vi "Handle LogRec.vi"(8 "error in":errorcluster, 10 "LogRecord":refnum<class "LogRecord.lvclass">, 11 "FileHandler in":refnum<class "FileHandler.lvclass">) -> (0 "error out":errorcluster, 3 "FileHandler out":refnum<class "FileHandler.lvclass">)   [LabVIEW 2024, in "hse-logger.lvlib" / "FileHandler.lvclass"]
doc: "Handles the incoming ``LogRecord`` object. If the level of the record is greater or equal to the level of the handler, then the record is written to the file. \n\n____\nHAMPEL SOFTWARE ENGINEERING v2.2.2 (2025-01-16 15:41)"
uses:
  <vilib>/Hampel Software Engineering/HSE Logger/Handler/FileHandler/FileHandler.lvclass
  <vilib>/Hampel Software Engineering/HSE Logger/LogRecord/LogRecord.lvclass
  <vilib>/Hampel Software Engineering/HSE Logger/LogRecord/LogRecord.lvclass/LogRecord.ctl
  <vilib>/Hampel Software Engineering/HSE Logger/Handler/FileHandler/FileHandler.lvclass/FileHandler.ctl
  <vilib>/Hampel Software Engineering/HSE Logger/Formatter/Formatter.lvclass
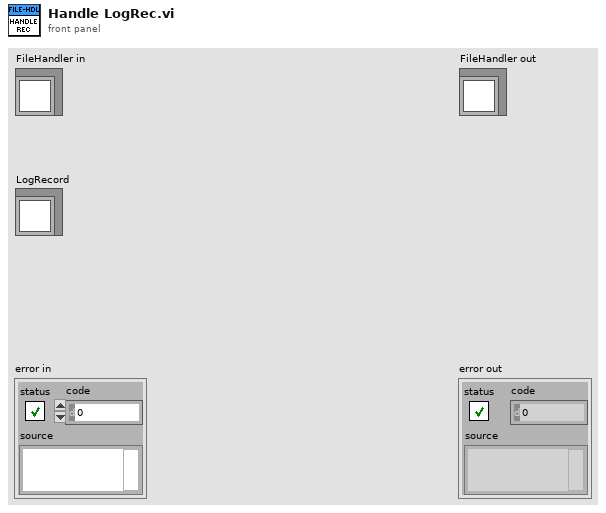
[diagram p1: front panel]
types:
  T1 = typedef "hse-logger.lvlib/LogLevel.ctl" = enum16{"DEBUG", "INFO", "WARNING", "ERROR", "CRITICAL"}
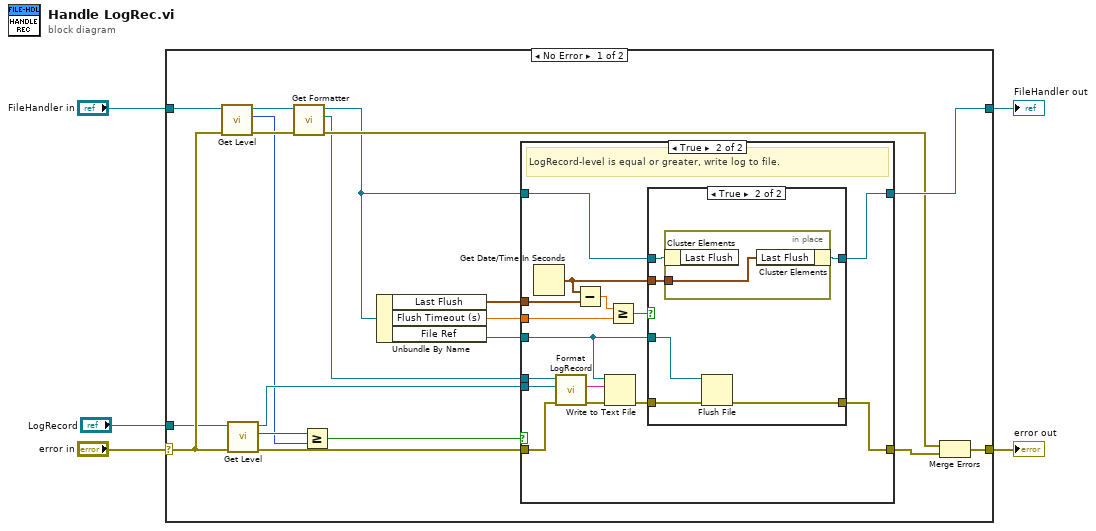
[diagram p0: block diagram]
diagram:
  n1 = case shown="No Error" "error in" {
    selector: "error in" -> [w23 w52]
    tunnel: [w13 w52] -> w4
    tunnel: [w10 w51] -> w2
    tunnel: "FileHandler in" -> [w20 w51]
    tunnel: "LogRecord" -> [w22 _]
    frame No Error {
      n2 = call-dynamic <vilib>:"Get Level.vi"("error in"=w23, "Handler in"=w20) -> ("error out"=w24:errorcluster, "Level"=w18:T1, "Handler out"=w8:refnum<class "FileHandler.lvclass">)  [unwired: 7 in]
      n3 = call <vilib>:"Get Level.vi"("error in"=w23, "LogRecord in"=w22) -> ("error out"=w16:errorcluster, "Level"=w19:T1, "LogRecord out"=w21:refnum<class "LogRecord.lvclass">)  [unwired: 7 in]
      n4 = call <vilib>:"Get Formatter.vi"("error in"=w24, "FileHandler"=w8) -> ("error out"=w9:errorcluster, "Formatter"=w6:refnum<class "Formatter.lvclass">, "FileHandler out"=w7:refnum<class "FileHandler.lvclass">)  [unwired: 7 in]
      n5 = Greater Or Equal?(x=w19, y=w18) -> (x >= y?=w17:bool)
      n6 = Unbundle By Name(w7) -> ("Last Flush"=w12:timestamp, "Flush Timeout (s)"=w11:dbl, "File Ref"=w15:refnum<file>)
      n7 = case shown="True" w17 {
        tunnel: w21 -> [_ w33]
        tunnel: w16 -> [w26 w32]
        tunnel: w15 -> [_ w29]
        tunnel: [w26 w35] -> w14
        tunnel: w12 -> [_ w41]
        tunnel: w11 -> [_ w39]
        tunnel: w7 -> [w25 w36]
        tunnel: [w25 w34] -> w10
        tunnel: w6 -> [_ w31]
        frame False {
          # "Do not write to file."
        }
        frame True {
          # "LogRecord-level is equal or greater, write log to file."
          n8 = Get Date/Time In Seconds() -> (seconds since 1Jan1904=w37:timestamp)
          n9 = call-dynamic "Format LogRecord.vi"("error in"=w32, "LogRecord"=w33, "Formatter in"=w31) -> ("error out"=w30:errorcluster, "LogLine"=w27:string)  [unwired: 7 in]
          n10 = Subtract(x=w37, y=w41) -> (x-y=w40:dbl)
          n11 = Write to Text File(file (use dialog)=w29, text=w27, error in=w30) -> (error out=w28:errorcluster)  [unwired: 1 in, 2 out]
          n12 = Greater Or Equal?(x=w40, y=w39) -> (x >= y?=w38:bool)
          n13 = case shown="True" w38 {
            tunnel: w28 -> [w42 w49]
            tunnel: w29 -> [_ w48]
            tunnel: w37 -> [_ w44]
            tunnel: w36 -> [w43 w46]
            tunnel: [w43 w45] -> w34
            tunnel: [w42 w47] -> w35
            frame False {
            }
            frame True {
              n14 = in-place {
                in-place-border: w44 -> [w50]
                n15 = in-place-cluster #1(w46) -> ()  [unwired: 1 out]
                n16 = in-place-cluster #1("Last Flush"=w50) -> (w45:refnum<class "FileHandler.lvclass">)
              }
              n17 = Flush File(refnum=w48, error in=w49) -> (error out=w47:errorcluster)  [unwired: 1 out]
            }
          }
        }
      }
      n18 = Merge Errors(w9, w14) -> (w13:errorcluster)
    }
    frame Error {
    }
  }
  "error out" <- w4
  "FileHandler out" <- w2
